vi "角度动态优化.vi"(7 "SENSOR":T1) -> (3 "OK？":bool)   [LabVIEW 2020]
panel:
  out "PROC":i32
  out "Temp1":dbl
  out "Temp":dbl
  out "S(%)":dbl
  out "P(%)":dbl
  out "error out":errorcluster caption="错误输出"
  in  "error in (no error)":errorcluster caption="错误输入（无错误）"
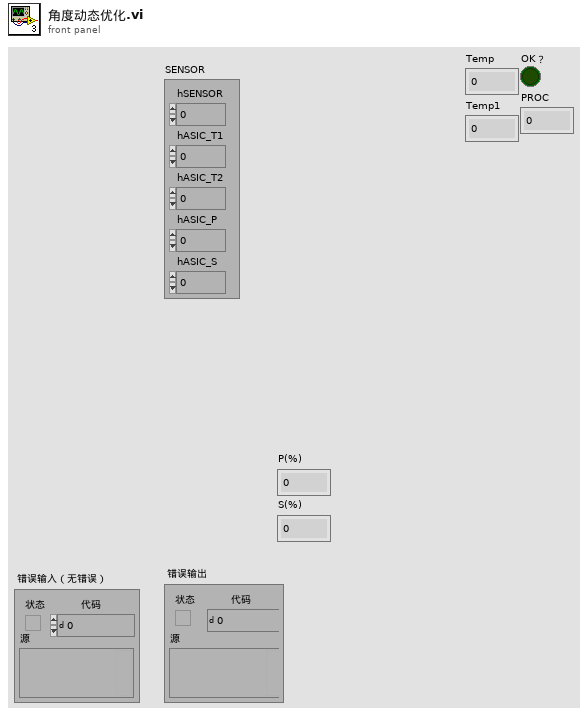
[diagram p1: front panel]
types:
  T1 = cluster{"hSENSOR":i32, "hASIC_T1":i32, "hASIC_T2":i32, "hASIC_P":i32, "hASIC_S":i32}
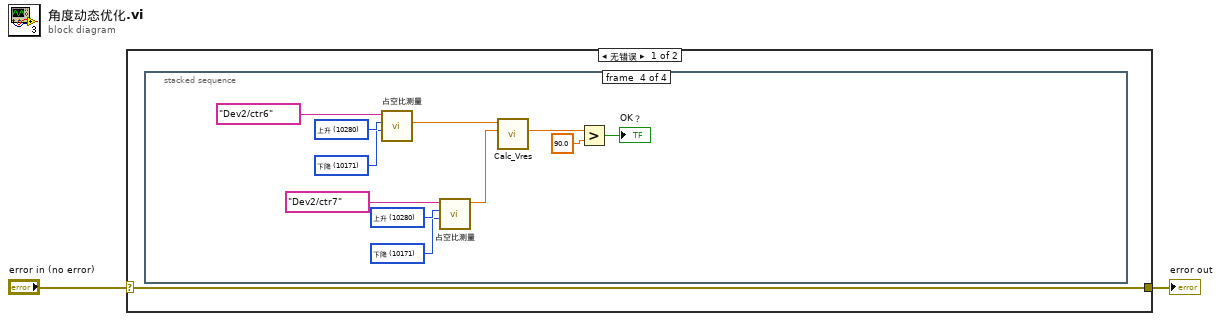
[diagram p0: block diagram]
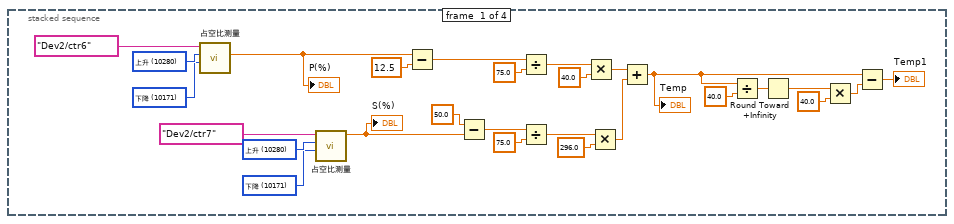
[diagram p2: hidden frame]
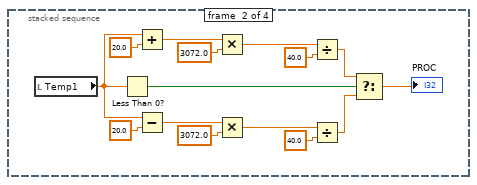
[diagram p3: hidden frame]
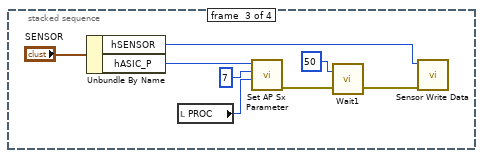
[diagram p4: hidden frame]
diagram:
  n1 = case shown="无错误" "error in (no error)" {
    selector: "error in (no error)" -> [w3 w65]
    tunnel: [w3 w65] -> w1
    frame No Error {
      n2 = stacked-sequence {
        frame #0 {
          w25 = 10171 items=["上升"=10280, "下降"=10171] ("starting edge2")
          w26 = 10280 items=["上升"=10280, "下降"=10171] ("starting edge1")
          w27 = 10171 items=["上升"=10280, "下降"=10171] ("starting edge2")
          w28 = 10280 items=["上升"=10280, "下降"=10171] ("starting edge1")
          n3 = call "占空比测量.vi"("计数器"=tag "Dev2/ctr6", "starting edge1"=w28, "starting edge2"=w27) -> ("占空比2(%)"=w24:dbl)  [unwired: 4 in, 3 out]
          "P(%)" <- w24
          n4 = call "占空比测量.vi"("计数器"=tag "Dev2/ctr7", "starting edge1"=w26, "starting edge2"=w25) -> ("占空比(%)"=w18:dbl)  [unwired: 4 in, 3 out]
          "S(%)" <- w18
          n5 = Subtract(x=w24, y=12.5) -> (x-y=w22:dbl)
          n6 = Subtract(x=50.0, y=w18) -> (x-y=w15:dbl)
          n7 = Divide(x=w22, y=75.0) -> (x/y=w20:dbl)
          n8 = Divide(x=w15, y=75.0) -> (x/y=w13:dbl)
          n9 = Multiply(x=w20, y=40.0) -> (x*y=w16:dbl)
          n10 = Multiply(x=w13, y=296.0) -> (x*y=w11:dbl)
          n11 = Add(x=w16, y=w11) -> (x+y=w10:dbl)
          "Temp" <- w10
          n12 = Divide(x=w10, y=40.0) -> (x/y=w8:dbl)
          n13 = Round Toward +Infinity(x=w8) -> (ceil(x): smallest int >= x=w7:dbl)
          n14 = Multiply(x=w7, y=40.0) -> (x*y=w5:dbl)
          n15 = Subtract(x=w10, y=w5) -> (x-y=→"Temp1":dbl)
        }
        frame #1 {
          n16 = local read "Temp1"() -> (w33:dbl)
          n17 = Less Than 0?(x=w33) -> (x < 0?=w45:bool)
          n18 = Add(x=w33, y=20.0) -> (x+y=w43:dbl)
          n19 = Subtract(x=w33, y=20.0) -> (x-y=w35:dbl)
          n20 = Multiply(x=w43, y=3072.0) -> (x*y=w41:dbl)
          n21 = Multiply(x=w35, y=3072.0) -> (x*y=w37:dbl)
          n22 = Divide(x=w41, y=40.0) -> (x/y=w39:dbl)
          n23 = Divide(x=w37, y=40.0) -> (x/y=w32:dbl)
          n24 = Select(t=w39, s=w45, f=w32) -> (s? t:f=→"PROC":dbl)
        }
        frame #2 {
          n25 = Unbundle By Name("SENSOR") -> ("hSENSOR"=w52:i32, "hASIC_P"=w53:i32)
          n26 = local read "PROC"() -> (w49:i32)
          n27 = call "Set AP Sx Parameter.vi"("para2"=w49, "asicBitsName"=7, "asicHandle"=w53) -> ("error out"=w51:errorcluster)  [unwired: 7 in, 1 out]
          n28 = call "Wait1.vi"("error in (no error)"=w51, "Wait（150ms）"=u32 50) -> ("error out"=w50:errorcluster)  [unwired: 1 in]
          n29 = call "Sensor Write Data.vi"("error in (no error)"=w50, "sensorHandle"=w52) -> ()  [unwired: 8 in, 2 out]
        }
        frame #3 {
          w62 = 10171 items=["上升"=10280, "下降"=10171] ("starting edge2")
          w63 = 10280 items=["上升"=10280, "下降"=10171] ("starting edge1")
          w59 = 10171 items=["上升"=10280, "下降"=10171] ("starting edge2")
          w60 = 10280 items=["上升"=10280, "下降"=10171] ("starting edge1")
          n30 = call "占空比测量.vi"("计数器"=tag "Dev2/ctr6", "starting edge1"=w60, "starting edge2"=w59) -> ("占空比2(%)"=w58:dbl)  [unwired: 4 in, 3 out]
          n31 = call "占空比测量.vi"("计数器"=tag "Dev2/ctr7", "starting edge1"=w63, "starting edge2"=w62) -> ("占空比(%)"=w57:dbl)  [unwired: 4 in, 3 out]
          n32 = call "Calc_Vres.vi"("S_Data in"=w57, "P_Data in"=w58) -> ("Vres"=w56:dbl)  [unwired: 7 in, 2 out]
          n33 = Greater?(x=w56, y=90.0) -> (0:→"OK？":bool)
        }
      }
    }
    frame Error {
    }
  }
  "error out" <- w1
